vi "Data Trends.vi"() -> ()   [LabVIEW 2013]
uses:
  <vilib>/Analysis/6fits.llb/Curve Fitting Criteria.ctl
  <vilib>/Analysis/6fits.llb/Prediction Interval (Exp).vi
  <vilib>/Analysis/1siggen.llb/Ramp Pattern by Delta.vi
  <vilib>/Analysis/polynomials.llb/1D Polynomial Evaluation (DBL).vi
  <vilib>/Analysis/NI_AALPro.lvlib
  <vilib>/Analysis/NI_AALBase.lvlib
panel:
  out "XY Graph 2":cluster{cluster{dbl, "Numeric":dbl}[]}[](graph)
  out "1-D Array of Real":dbl[](array[numeric])
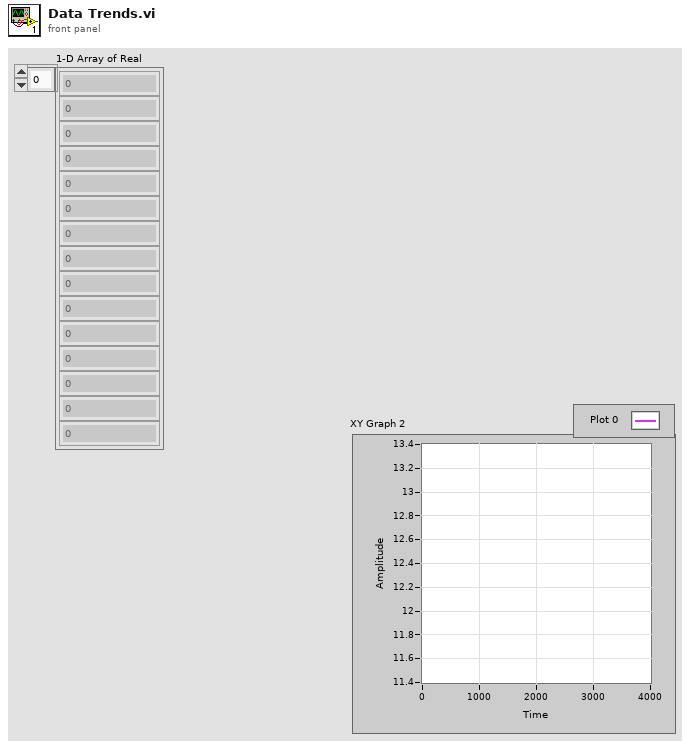
[diagram p1: front panel]
types:
  T1 = typedef "NI_AALPro.lvlib/Curve Fitting Criteria.ctl" = u16
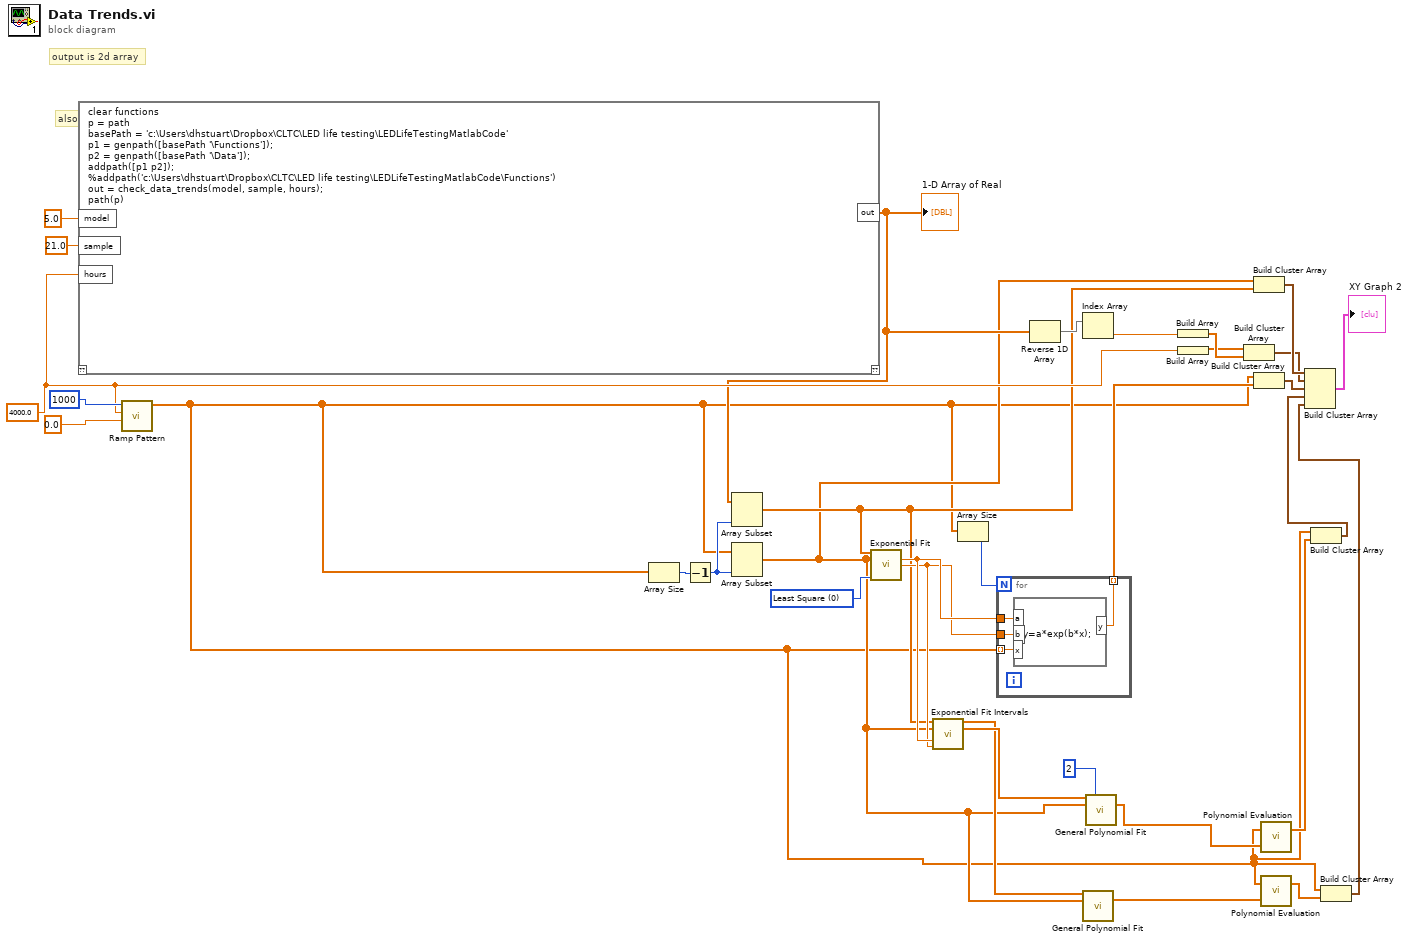
[diagram p0: block diagram]
diagram:
  w29 = T1 0 items=["Least Square", "Least Absolute Residual", "Bisquare"] ("method")
  w18 = 4000.0 ("Real")
  # "also output an array of data names"
  # "output is 2d array"
  n1 = script code="clear functions\np = path\nbasePath = 'c:\\Users\\dhstuart\\Dropbox\\CLTC\\LED life testing\\LEDLifeTestingMatlabCode'\np1 = genpath([basePath '\\Functions']);\np2 = genpath([basePath '\\Data']);\naddpath([p1 p2]);\n%addpath('c:\\Users\\dhstuart\\Dropbox\\CLTC\\LED life testing\\LEDLifeTestingMatlabCode\\Functions')\nout = check_data_trends(model, sample, hours);\npath(p)"("model"=5.0 ("Real"), "sample"=21.0 ("Real"), "hours"=w18) -> ("out"=w15:dbl[])  [unwired: 1 in, 1 out]
  "1-D Array of Real" <- w15
  n2 = call-poly <vilib>:"Ramp Pattern.vi"("start"=0.0, "end"=w18, "delta"=1000 ("samples")) -> ("Ramp Pattern"=w1:dbl[])  [unwired: 6 in, 2 out]
  n3 = Array Size(array=w1) -> (size(s)=w26:i32)
  n4 = Decrement(x=w26) -> (x-1=w25:i32)
  n5 = Array Subset(array=w15, length=w25) -> (w12:dbl[])  [unwired: 1 in]
  n6 = Array Subset(array=w1, length=w25) -> (w6:dbl[])  [unwired: 1 in]
  n7 = call <vilib>:"Exponential Fit.vi"("Y"=w12, "X"=w6, "method"=w29) -> ("amplitude"=w14:dbl, "damping"=w13:dbl)  [unwired: 7 in, 4 out]
  n8 = call-poly <vilib>:"Exponential Fit Intervals.vi"("Y"=w12, "X"=w6, "amplitude"=w14, "damping"=w13) -> ("Upper Bound"=w7:dbl[], "Lower Bound"=w11:dbl[])  [unwired: 9 in, 1 out]
  n9 = Array Size(array=w1) -> (size(s)=w24:i32)
  n10 = for {
    N: w24 -> [_]
    tunnel: w14 -> [w37]
    tunnel: w13 -> [w36]
    tunnel: w1 -> [w35] mode=indexing
    tunnel: [w34] -> w23 mode=indexing
    n11 = formula code="y=a*exp(b*x);"("a"=w37, "b"=w36, "x"=w35) -> ("y"=w34:dbl)
  }
  n12 = Reverse 1D Array(array=w15) -> (reversed array=w16:dbl[])
  n13 = Index Array(array=w16) -> (element=w21:dbl)  [unwired: 1 in]
  n14 = call <vilib>:"General Polynomial Fit.vi"("Y"=w7, "X"=w6) -> ("Polynomial Coefficients"=w4:dbl[])  [unwired: 10 in, 3 out]
  n15 = call <vilib>:"General Polynomial Fit.vi"("Y"=w11, "polynomial order"=2, "X"=w6) -> ("Polynomial Coefficients"=w8:dbl[])  [unwired: 9 in, 3 out]
  n16 = Build Array(w21) -> (w20:dbl[])
  n17 = Build Array(w18) -> (w19:dbl[])
  n18 = Build Cluster Array(w19, w20) -> (w17:cluster{"Real":dbl, dbl}[])
  n19 = Build Cluster Array(w6, w12) -> (w28:cluster{dbl, dbl}[])
  n20 = Build Cluster Array(w1, w23) -> (w22:cluster{dbl, "y":dbl}[])
  n21 = call-poly <vilib>:"Polynomial Evaluation.vi"("P(x)"=w8, "A"=w1) -> ("P(A)"=w10:dbl[])  [unwired: 1 out]
  n22 = call-poly <vilib>:"Polynomial Evaluation.vi"("P(x)"=w4, "A"=w1) -> ("P(A)"=w3:dbl[])  [unwired: 1 out]
  n23 = Build Cluster Array(w1, w10) -> (w5:cluster{dbl, "p(x)":dbl}[])
  n24 = Build Cluster Array(w1, w3) -> (w2:cluster{dbl, "p(x)":dbl}[])
  n25 = Build Cluster Array(w28, w17, w22, w5, w2) -> (→"XY Graph 2":cluster{cluster{"Real":dbl, "p(x)":dbl}[]}[])
